vi "Set Controler Scheme.vi"(8 "error in (no error)":errorcluster, 10 "Configuration":T4, 11 "JoystickDevRef":T1) -> (0 "error out":errorcluster, 2 "Control Values":T3, 3 "JoystickDevRef":T1)   [LabVIEW 2016]
uses:
  <vilib>/Rock Robotics/WPI/Joystick/WPI_JoystickDevRef.ctl
  <vilib>/Rock Robotics/WPI/Joystick/WPI_JoystickDeviceEnum.ctl
  <vilib>/Rock Robotics/Network Tables/NT Write Numeric Array.vi
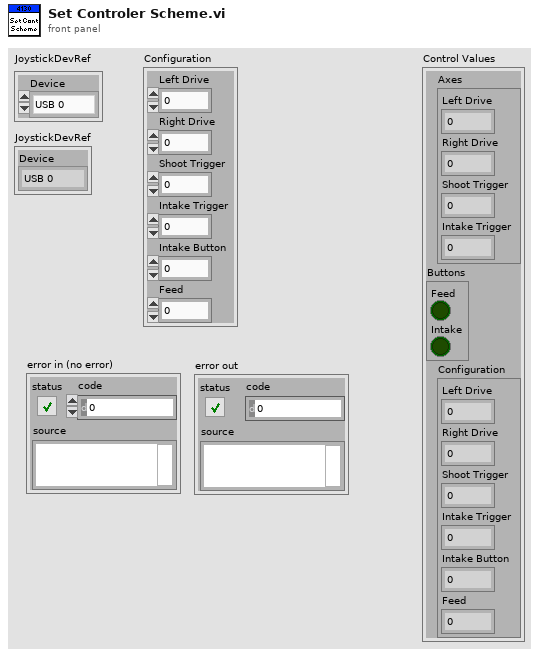
[diagram p1: front panel]
types:
  T1 = typedef "WPI_JoystickDevRef.ctl" = cluster{"Device":T2}
  T2 = typedef "WPI_JoystickDeviceEnum.ctl" = enum16{"USB 0", "USB 1", "USB 2", "USB 3", "USB 4", "USB 5"}
  T3 = cluster{"Axes":cluster{"Left Drive":dbl, "Right Drive":dbl, "Shoot Trigger":dbl, "Intake Trigger":dbl}, "Buttons":cluster{"Feed":bool, "Intake":bool}, "Configuration":cluster{"Left Drive":i32, "Right Drive":i32, "Shoot Trigger":i32, "Intake Trigger":i32, "Intake Button":i32, "Feed":i32}}
  T4 = cluster{"Left Drive":i32, "Right Drive":i32, "Shoot Trigger":i32, "Intake Trigger":i32, "Intake Button":i32, "Feed":i32}
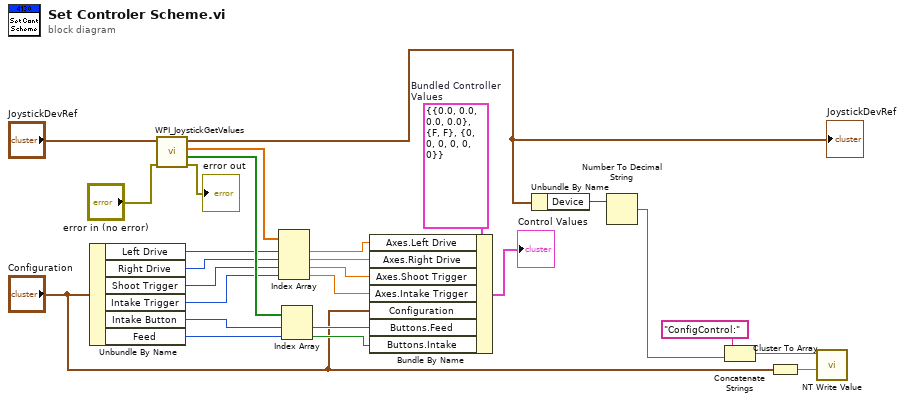
[diagram p0: block diagram]
diagram:
  w26 = T3 {"Axes"={"Left Drive"=0.0, "Right Drive"=0.0, "Shoot Trigger"=0.0, "Intake Trigger"=0.0}, "Buttons"={"Feed"=FALSE, "Intake"=FALSE}, "Configuration"={"Left Drive"=0, "Right Drive"=0, "Shoot Trigger"=0, "Intake Trigger"=0, "Intake Button"=0, "Feed"=0}}  # Bundled Controller Values
  n1 = Unbundle By Name("Configuration") -> ("Left Drive"=w13:i32, "Right Drive"=w12:i32, "Shoot Trigger"=w8:i32, "Intake Trigger"=w9:i32, "Intake Button"=w10:i32, "Feed"=w11:i32)
  n2 = call <vilib>:"WPI_JoystickGetValues.vi"("error in (no error)"="error in (no error)", "JoystickDevRef"="JoystickDevRef") -> ("error out"=→"error out":errorcluster, "Buttons"=w18:bool[], "Axes"=w19:dbl[], "JoystickDevRef"=w3:T1)  [unwired: 5 in, 1 out]
  "JoystickDevRef" <- w3
  n3 = Index Array(array=w19, index #1=w13, index #2=w12, index #3=w8, index #4=w9) -> (element #1=w25:dbl, element #2=w24:dbl, element #3=w23:dbl, element #4=w22:dbl)
  n4 = Index Array(array=w18, index #1=w10, index #2=w11) -> (element #1=w21:bool, element #2=w20:bool)
  n5 = Bundle By Name(cluster=w26, "Axes.Left Drive"=w25, "Axes.Right Drive"=w24, "Axes.Shoot Trigger"=w23, "Axes.Intake Trigger"=w22, "Configuration"="Configuration", "Buttons.Feed"=w21, "Buttons.Intake"=w20) -> (→"Control Values":T3)
  n6 = Unbundle By Name(w3) -> ("Device"=w6:T2)
  n7 = Number To Decimal String(number=w6) -> (decimal integer string=w4:string)  [unwired: 1 in]
  n8 = Concatenate Strings("ConfigControl:", w4) -> (w2:string)
  n9 = Cluster To Array(cluster="Configuration") -> (array=w7:i32[])
  n10 = call-poly <vilib>:"NT Write Value.vi"("Numeric Array"=w7, "Name"=w2) -> ()  [unwired: 9 in, 1 out]
